vi "Vision.vi"(5 "Minimum Confidence":dbl=0.15) -> (1 "ball detected":bool, 4 "Confidence":dbl, 6 "y Coordinate of Ball":dbl, 8 "x Coordinate of Ball":dbl, 10 "z Coordinate of Goal":dbl, 12 "Goal Detected":bool, 14 "Goal Angle (radians 0=right)":dbl, 15 "Goal Distance":dbl)   [LabVIEW 2015]
uses:
  <vilib>/Analysis/Matrix/Datatypes/RealMatrix.ctl
  Team900-VIs/labview-zmq/socket_type.ctl
  Team900-VIs/labview-zmq/socket_options.ctl
  <vilib>/Analysis/Matrix/Numeric/Conversions/Array To Matrix - RA2.vi
  <vilib>/Analysis/Matrix/NI_Matrix.lvlib
  Team900-VIs/labview-zmq/zmq_socket.lvclass
  Team900-VIs/labview-zmq/zmq_context.lvclass
  Team900-VIs/labview-zmq/zeromq.lvlib
  <vilib>/Rock Robotics/Network Tables/NT Read Number.vi
panel:
  out "data 2":string
  in  "Max height":dbl
  out "Real Matrix":T1
  out "data":string
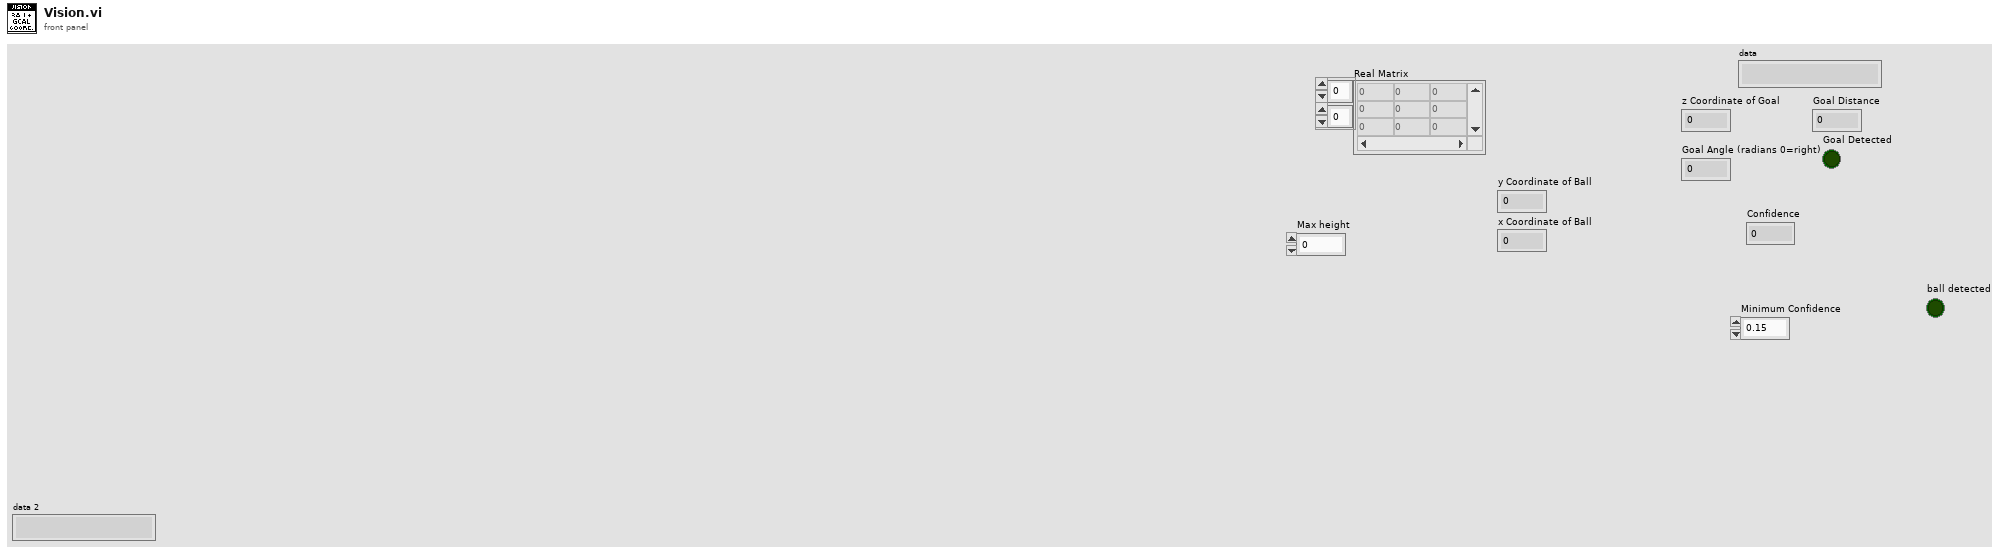
[diagram p1: front panel]
types:
  T1 = typedef "NI_Matrix.lvlib/RealMatrix.ctl" = dbl[][]
  T2 = typedef "zeromq.lvlib/socket_options.ctl" = enum8{"NONE", "ZMQ_HWM", "<2>", "ZMQ_SWAP", "ZMQ_AFFINITY", "ZMQ_IDENTITY", "ZMQ_SUBSCRIBE", "ZMQ_UNSUBSCRIBE", "ZMQ_RATE", "ZMQ_RECOVERY_IVL", "ZMQ_MCAST_LOOP", "ZMQ_SNDBUF", "ZMQ_RCVBUF", "ZMQ_RCVMORE", "ZMQ_FD", "ZMQ_EVENTS", "ZMQ_TYPE", "ZMQ_LINGER", "ZMQ_RECONNECT_IVL", "ZMQ_BACKLOG", "ZMQ_RECOVERY_IVL_MSEC", "ZMQ_RECONNECT_IVL_MAX", "ZMQ_MAXMSGSIZE", "ZMQ_SNDHWM", "ZMQ_RCVHWM", "ZMQ_MULTICAST_HOPS", "<26>", "ZMQ_RCVTIMEO", "ZMQ_SNDTIMEO", "<29>", "<30>", "ZMQ_IPV4ONLY", "ZMQ_LAST_ENDPOINT", "ZMQ_ROUTER_MANDATORY", "ZMQ_TCP_KEEPALIVE", "ZMQ_TCP_KEEPALIVE_CNT", "ZMQ_TCP_KEEPALIVE_IDLE", "ZMQ_TCP_KEEPALIVE_INTVL", "ZMQ_TCP_ACCEPT_FILTER", "ZMQ_DELAY_ATTACH_ON_CONNECT", "ZMQ_XPUB_VERBOSE"}
  T3 = typedef "zeromq.lvlib/socket_type.ctl" = enum8{"ZMQ_PAIR", "ZMQ_PUB", "ZMQ_SUB", "ZMQ_REQ", "ZMQ_REP", "ZMQ_DEALER", "ZMQ_ROUTER", "ZMQ_PULL", "ZMQ_PUSH", "ZMQ_XPUB", "ZMQ_XSUB"}
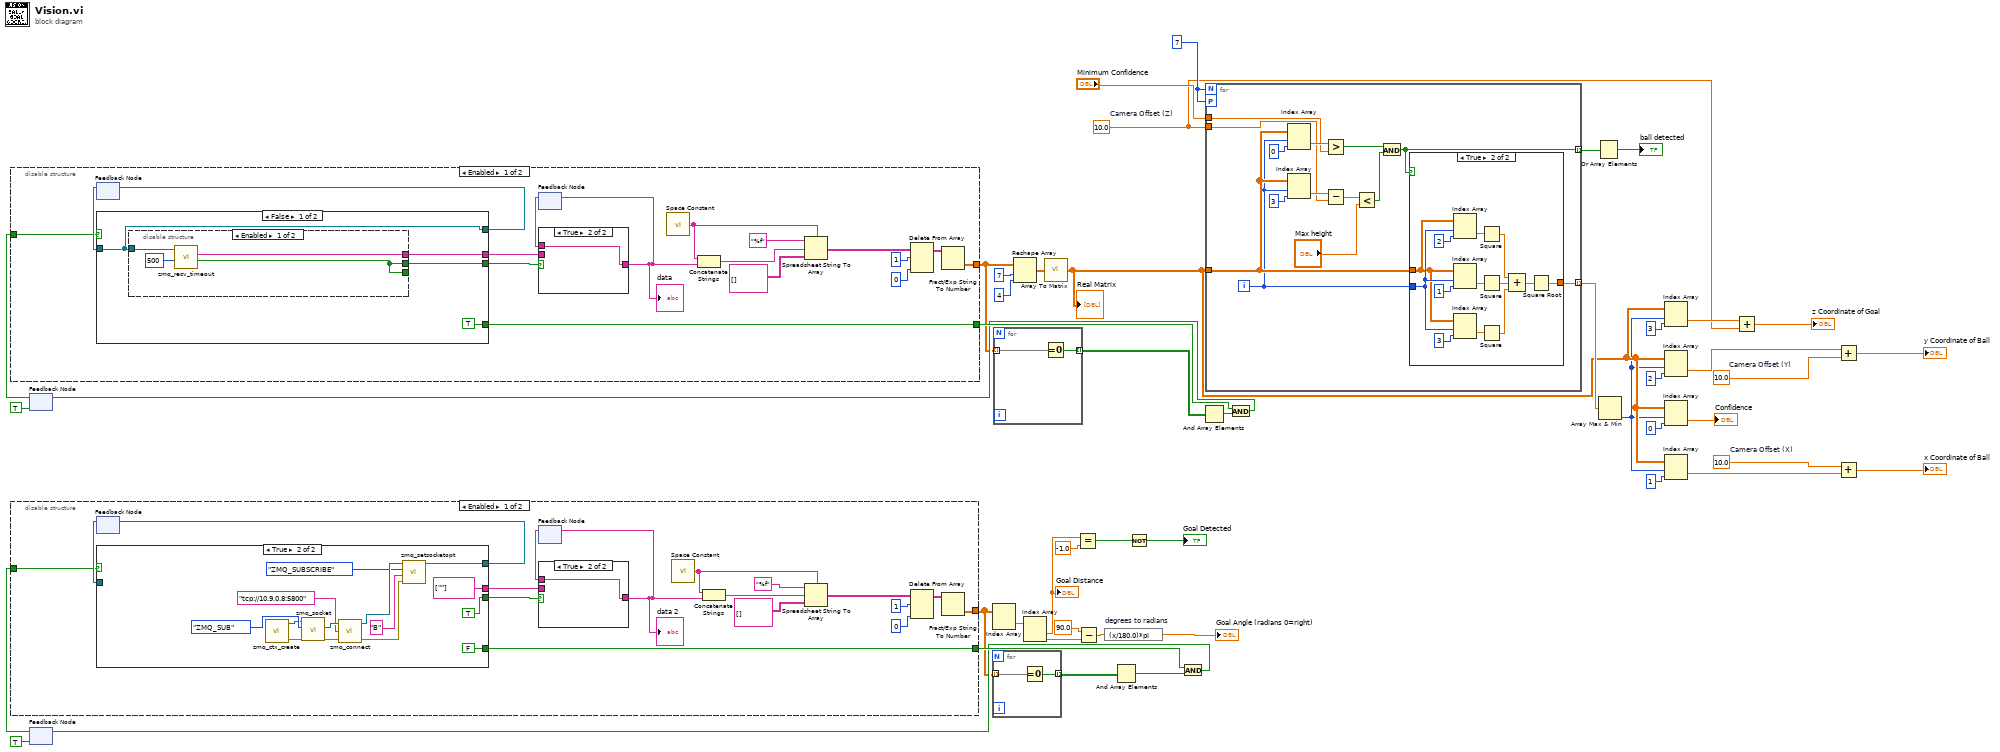
[diagram p0: block diagram]
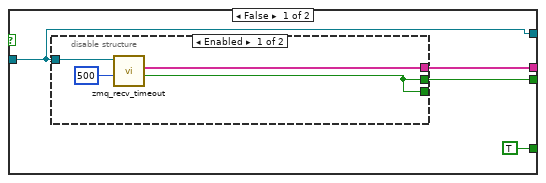
[diagram p2: hidden frame]
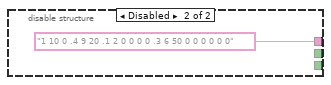
[diagram p3: hidden frame]
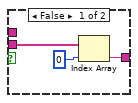
[diagram p4: hidden frame]
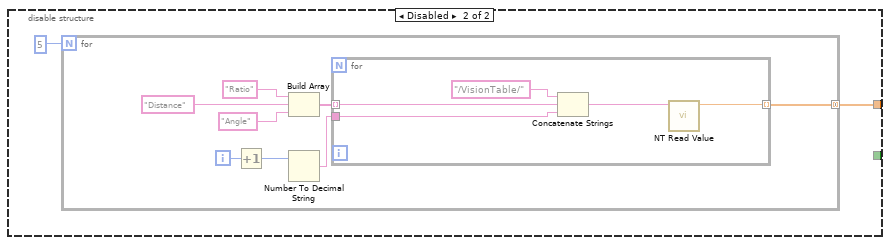
[diagram p5: hidden frame]
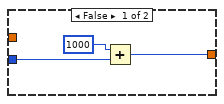
[diagram p6: hidden frame]
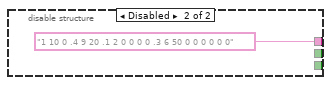
[diagram p7: hidden frame]
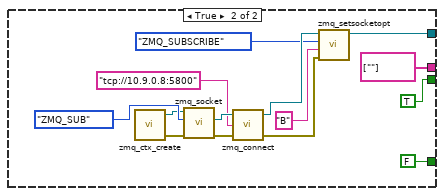
[diagram p8: hidden frame]
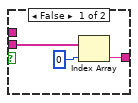
[diagram p9: hidden frame]
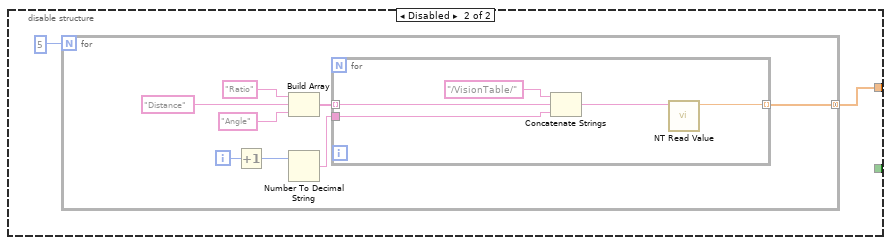
[diagram p10: hidden frame]
diagram:
  w20 = 10.0  # Camera Offset (Y)
  w21 = 10.0  # Camera Offset (X)
  w24 = 10.0  # Camera Offset (Z)
  w44 = 7
  n1 = feedback #1(TRUE) -> (w12:bool)
  n2 = disable-structure shown="Enabled" {
    disable-tunnel: [w58 w93] -> w32
    disable-tunnel: w12 -> [w48 _]
    disable-tunnel: [w49 _] -> w34
    frame Enabled {
      n3 = feedback #2() -> (w50:refnum<class "zmq_socket.lvclass">)  [unwired: 1 in]
      n4 = case shown="False" w48 {
        tunnel: [w68 string[] [""] ("parts")] -> w53
        tunnel: [w67 TRUE ("timeout?")] -> w52
        tunnel: w50 -> [w66 _]
        tunnel: [w66 w75] -> w51
        tunnel: [TRUE FALSE] -> w49
        frame False {
          n5 = disable-structure shown="Enabled" {
            disable-tunnel: [w72 "1 10 0 .4 9 20 .1 2 0 0 0 0 .3 6 50 0 0 0 0 0 0"] -> w68
            disable-tunnel: [w70 _] -> w67
            disable-tunnel: [w70 _] -> _
            disable-tunnel: w66 -> [w69 _]
            frame Enabled {
              n6 = call "zmq_recv_timeout.vi"("timeout (ms)"=u32 500, "socket in"=w69) -> ("timeout?"=w70:bool, "parts"=w72:string[])  [unwired: 2 in, 2 out]
            }
            frame Disabled {
            }
          }
        }
        frame True {
          n7 = call "zmq_ctx_create.vi"() -> ("error out"=w83:errorcluster, "context out"=w86:refnum<class "zmq_context.lvclass">)  [unwired: 4 in]
          n8 = call "zmq_socket.vi"("error in"=w83, "socket type"=socket_type."ZMQ_SUB", "context in"=w86) -> ("error out"=w80:errorcluster, "socket out"=w85:refnum<class "zmq_socket.lvclass">)  [unwired: 2 in, 1 out]
          n9 = call "zmq_connect.vi"("error in"=w80, "endpoint"="tcp://10.9.0.8:5800" ("Endpoint"), "socket in"=w85) -> ("error out"=w81:errorcluster, "socket out"=w82:refnum<class "zmq_socket.lvclass">)  [unwired: 1 in]
          n10 = call "zmq_setsocketopt.vi"("error in"=w81, "value"="B", "option"=socket_options."ZMQ_SUBSCRIBE", "socket in"=w82) -> ("socket out"=w75:refnum<class "zmq_socket.lvclass">)  [unwired: 2 in, 1 out]
        }
      }
      n11 = feedback-in #2(w51) -> ()
      n12 = feedback #3() -> (w54:string)  [unwired: 1 in]
      n13 = case shown="True" w52 {
        tunnel: w53 -> [w90 _]
        tunnel: [w88 w91] -> w55
        tunnel: w54 -> [_ w91]
        frame False {
          n14 = Index Array(array=w90, index=0) -> (element=w88:string)
        }
        frame True {
        }
      }
      "data" <- w55
      n15 = feedback-in #3(w55) -> ()
      n16 = call <vilib>:"Space Constant.vi"() -> ("String"=w56:string)
      n17 = Concatenate Strings(w56, w55) -> (w57:string)
      n18 = Spreadsheet String To Array(delimiter (Tab)=w56, format string="%f", spreadsheet string=w57, array type (2D Dbl)=string[][] [] ("Array")) -> (array=w59:string[][])
      n19 = Delete From Array(array=w59, length=1, index (col)=0 ("disabled index (col)")) -> (array with subset deleted=w60:string[][])  [unwired: 1 in, 1 out]
      n20 = Fract/Exp String To Number(string=w60) -> (number=w58:dbl[][])  [unwired: 4 out]
    }
    frame Disabled {
      n21 = for {
        N: 5 -> [_]
        tunnel: [w101] -> w93 mode=concatenating
        i -> [w96]
        n22 = Increment(x=w96) -> (x+1=w95:i32)
        n23 = Build Array("Ratio" ("element"), "Distance" ("element"), "Angle") -> (w97:string[])
        n24 = Number To Decimal String(number=w95) -> (decimal integer string=w94:string)  [unwired: 1 in]
        n25 = for {
          tunnel: [w105] -> w101 mode=indexing
          tunnel: w97 -> [w104] mode=indexing
          tunnel: w94 -> [w102]
          n26 = Concatenate Strings("/VisionTable/" ("string"), w104, w102) -> (w106:string)
          n27 = call-poly <vilib>:"NT Read Value.vi"("Name"=w106) -> ("Numeric"=w105:dbl)  [unwired: 9 in, 1 out]
        }
      }
    }
  }
  n28 = feedback #4(TRUE) -> (w11:bool)
  n29 = disable-structure shown="Enabled" {
    disable-tunnel: [w117 w152] -> w10
    disable-tunnel: w11 -> [w107 _]
    disable-tunnel: [w108 _] -> w15
    frame Enabled {
      n30 = feedback #5() -> (w109:refnum<class "zmq_socket.lvclass">)  [unwired: 1 in]
      n31 = case shown="True" w107 {
        tunnel: [w127 string[] [""] ("parts")] -> w112
        tunnel: [w126 TRUE ("timeout?")] -> w111
        tunnel: w109 -> [w125 _]
        tunnel: [w125 w134] -> w110
        tunnel: [TRUE FALSE] -> w108
        frame False {
          n32 = disable-structure shown="Enabled" {
            disable-tunnel: [w131 "1 10 0 .4 9 20 .1 2 0 0 0 0 .3 6 50 0 0 0 0 0 0"] -> w127
            disable-tunnel: [w129 _] -> w126
            disable-tunnel: [w129 _] -> _
            disable-tunnel: w125 -> [w128 _]
            frame Enabled {
              n33 = call "zmq_recv_timeout.vi"("timeout (ms)"=u32 500, "socket in"=w128) -> ("timeout?"=w129:bool, "parts"=w131:string[])  [unwired: 2 in, 2 out]
            }
            frame Disabled {
            }
          }
        }
        frame True {
          n34 = call "zmq_ctx_create.vi"() -> ("error out"=w142:errorcluster, "context out"=w145:refnum<class "zmq_context.lvclass">)  [unwired: 4 in]
          n35 = call "zmq_socket.vi"("error in"=w142, "socket type"=socket_type."ZMQ_SUB", "context in"=w145) -> ("error out"=w139:errorcluster, "socket out"=w144:refnum<class "zmq_socket.lvclass">)  [unwired: 2 in, 1 out]
          n36 = call "zmq_connect.vi"("error in"=w139, "endpoint"="tcp://10.9.0.8:5800" ("Endpoint"), "socket in"=w144) -> ("error out"=w140:errorcluster, "socket out"=w141:refnum<class "zmq_socket.lvclass">)  [unwired: 1 in]
          n37 = call "zmq_setsocketopt.vi"("error in"=w140, "value"="B", "option"=socket_options."ZMQ_SUBSCRIBE", "socket in"=w141) -> ("socket out"=w134:refnum<class "zmq_socket.lvclass">)  [unwired: 2 in, 1 out]
        }
      }
      n38 = feedback-in #5(w110) -> ()
      n39 = feedback #6() -> (w113:string)  [unwired: 1 in]
      n40 = case shown="True" w111 {
        tunnel: w112 -> [w149 _]
        tunnel: [w147 w150] -> w114
        tunnel: w113 -> [_ w150]
        frame False {
          n41 = Index Array(array=w149, index=0) -> (element=w147:string)
        }
        frame True {
        }
      }
      "data 2" <- w114
      n42 = feedback-in #6(w114) -> ()
      n43 = call <vilib>:"Space Constant.vi"() -> ("String"=w115:string)
      n44 = Concatenate Strings(w115, w114) -> (w116:string)
      n45 = Spreadsheet String To Array(delimiter (Tab)=w115, format string="%f", spreadsheet string=w116, array type (2D Dbl)=string[][] [] ("Array")) -> (array=w118:string[][])
      n46 = Delete From Array(array=w118, length=1, index (col)=0 ("disabled index (col)")) -> (array with subset deleted=w119:string[][])  [unwired: 1 in, 1 out]
      n47 = Fract/Exp String To Number(string=w119) -> (number=w117:dbl[][])  [unwired: 4 out]
    }
    frame Disabled {
      n48 = for {
        N: 5 -> [_]
        tunnel: [w160] -> w152 mode=concatenating
        i -> [w155]
        n49 = Increment(x=w155) -> (x+1=w154:i32)
        n50 = Build Array("Ratio" ("element"), "Distance" ("element"), "Angle") -> (w156:string[])
        n51 = Number To Decimal String(number=w154) -> (decimal integer string=w153:string)  [unwired: 1 in]
        n52 = for {
          tunnel: [w164] -> w160 mode=indexing
          tunnel: w156 -> [w163] mode=indexing
          tunnel: w153 -> [w161]
          n53 = Concatenate Strings("/VisionTable/" ("string"), w163, w161) -> (w165:string)
          n54 = call-poly <vilib>:"NT Read Value.vi"("Name"=w165) -> ("Numeric"=w164:dbl)  [unwired: 9 in, 1 out]
        }
      }
    }
  }
  n55 = Index Array(array=w10) -> (element=w9:dbl[])  [unwired: 2 in]
  n56 = for {
    tunnel: w10 -> [w167] mode=indexing
    tunnel: [w166] -> w17 mode=indexing
    n57 = Equal To 0?(x=w167) -> (x = 0?=w166:bool[])
  }
  n58 = for {
    tunnel: w32 -> [w169] mode=indexing
    tunnel: [w168] -> w36 mode=indexing
    n59 = Equal To 0?(x=w169) -> (x = 0?=w168:bool[])
  }
  n60 = Reshape Array(w32, 7 ("dimension size"), 4 ("dimension size")) -> (w45:dbl[][])
  n61 = Index Array(array=w9) -> (element #1=w4:dbl, element #2=w8:dbl)  [unwired: 2 in]
  "Goal Distance" <- w4
  n62 = call-poly <vilib>:"Array To Matrix.vi"("Real 2D Array"=w45) -> ("Real Matrix"=w30:T1)
  "Real Matrix" <- w30
  n63 = Equal?(x=w4, y=-1.0) -> (x = y?=w2:bool)
  n64 = Subtract(x=90.0, y=w8) -> (x-y=w6:dbl)
  n65 = expression code="(x/180.0)*pi" "degrees to radians"(w6) -> (→"Goal Angle (radians 0=right)":dbl)
  n66 = And Array Elements(Boolean array=w17) -> (logical AND=w16:bool)
  n67 = Not(x=w2) -> (.not. x?=→"Goal Detected":bool)
  n68 = And(x=w15, y=w16) -> (x .and. y?=w14:bool)
  n69 = feedback-in #4(w14) -> ()
  n70 = And Array Elements(Boolean array=w36) -> (logical AND=w35:bool)
  n71 = for {
    N: w44 -> [_]
    workers-P: w44 -> [_]
    tunnel: w30 -> [w178]
    tunnel: "Minimum Confidence" -> [w182]
    tunnel: [w180] -> w42 mode=indexing
    tunnel: [w170] -> w18 mode=indexing
    tunnel: w24 -> [w174]
    i -> [w177]
    n72 = Index Array(array=w178, index (row)=w177, index (col)=0) -> (element=w183:dbl)
    n73 = Index Array(array=w178, index (row)=w177, index (col)=3) -> (element=w176:dbl)
    n74 = Greater?(x=w183, y=w182) -> (0:w172:bool)
    n75 = Subtract(x=w176, y=w174) -> (x-y=w175:dbl)
    n76 = Less?(x=w175, y="Max height") -> (x < y?=w171:bool)
    n77 = And(x=w172, y=w171) -> (x .and. y?=w170:bool)
    n78 = case shown="True" w170 {
      tunnel: w177 -> [w184 w196]
      tunnel: w178 -> [_ w195]
      tunnel: [w185 w187] -> w180
      frame False {
        n79 = Add(x=1000, y=w184) -> (x+y=w185:i32)
      }
      frame True {
        n80 = Index Array(array=w195, index (row)=w196, index (col)=2) -> (element=w194:dbl)
        n81 = Index Array(array=w195, index (row)=w196, index (col)=1) -> (element=w192:dbl)
        n82 = Index Array(array=w195, index (row)=w196, index (col)=3) -> (element=w193:dbl)
        n83 = Square(x=w194) -> (x^2=w191:dbl)
        n84 = Square(x=w192) -> (x^2=w190:dbl)
        n85 = Square(x=w193) -> (x^2=w189:dbl)
        n86 = Compound Arithmetic op=ADD(w191, w190, w189) -> (w188:dbl)
        n87 = Square Root(x=w188) -> (sqrt(x)=w187:dbl)
      }
    }
  }
  n88 = And(x=w34, y=w35) -> (x .and. y?=w33:bool)
  n89 = feedback-in #1(w33) -> ()
  n90 = Or Array Elements(Boolean array=w18) -> (logical OR=→"ball detected":bool)
  n91 = Array Max & Min(array=w42) -> (min index (indices)=w29:i32)  [unwired: 3 out]
  n92 = Index Array(array=w30, index (row)=w29, index (col)=3) -> (element=w26:dbl)
  n93 = Index Array(array=w30, index (row)=w29, index (col)=2) -> (element=w27:dbl)
  n94 = Index Array(array=w30, index (row)=w29, index (col)=0) -> (element=→"Confidence":dbl)
  n95 = Index Array(array=w30, index (row)=w29, index (col)=1) -> (element=w28:dbl)
  n96 = Add(x=w26, y=w24) -> (x+y=→"z Coordinate of Goal":dbl)
  n97 = Add(x=w27, y=w20) -> (x+y=→"y Coordinate of Ball":dbl)
  n98 = Add(x=w21, y=w28) -> (x+y=→"x Coordinate of Ball":dbl)
